vi "FTW-JSON-Core-Serialize.vi"(0 "JSON Object":i64 format="%016x", 5 "Encoding Flags":i64 format="%016x", 11 "error in":errorcluster) -> (4 "JSON Object":i64 format="%016x", 6 "JSON String (UTF-8)":string, 15 "error out":errorcluster)   [LabVIEW 2013, in "FTW-JSON.lvclass"]
uses:
  FTW-JSON.lvclass
panel:
  # "Inputs"
  # "Outputs"
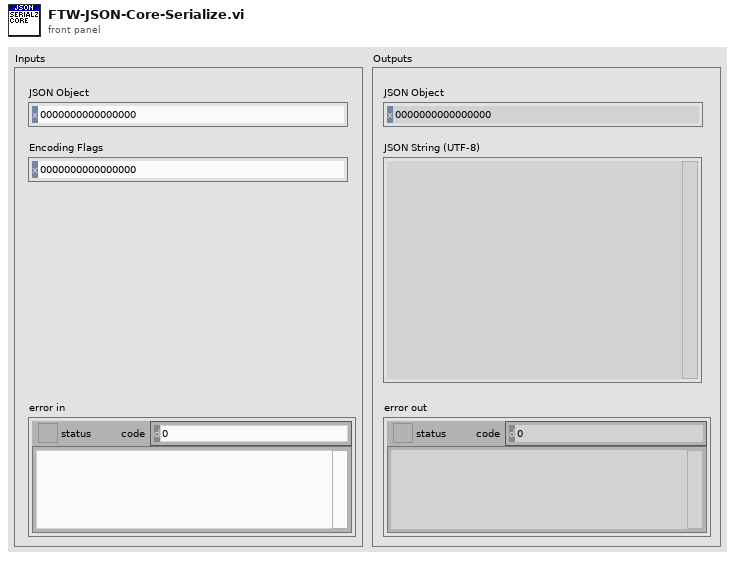
[diagram p1: front panel]
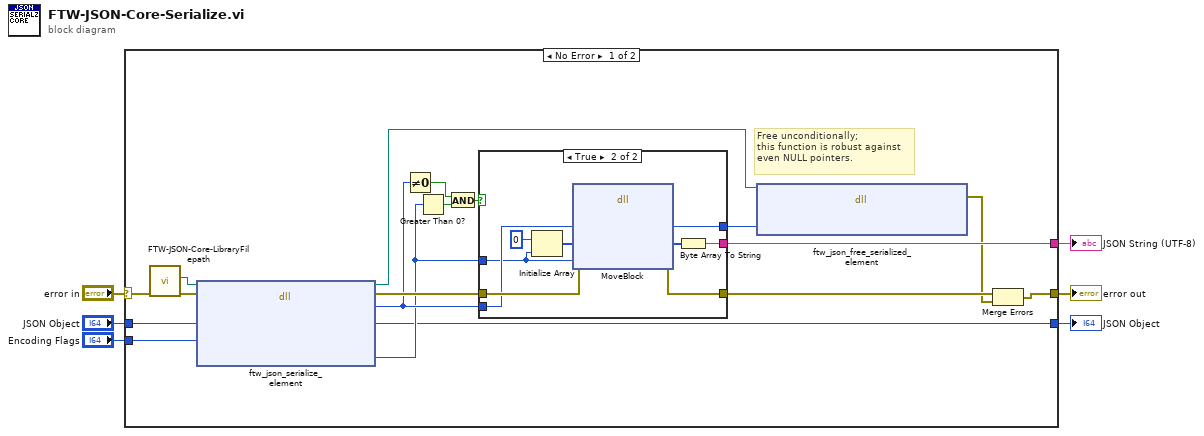
[diagram p0: block diagram]
diagram:
  n1 = case shown="No Error" "error in" {
    selector: "error in" -> [w24 w37]
    tunnel: [w23 w37] -> w6
    tunnel: [w7 w36] -> w4
    tunnel: "JSON Object" -> [w9 w36]
    tunnel: [w22 _] -> w2
    tunnel: "Encoding Flags" -> [w8 _]
    frame No Error {
      # "Free unconditionally;\nthis function is robust against\neven NULL pointers."
      n2 = call "FTW-JSON-Core-LibraryFilepath.vi"("error in"=w24) -> ("error out"=w21:errorcluster, "JSON Library Filepath"=w20:path)  [unwired: 9 in]
      n3 = dll-call lib="?" fn="ftw_json_serialize_element"(path in=w20, error in=w21, "JSON Object Pointer"=w9, "Flags"=w8) -> (path out=w10:path, error out=w19:errorcluster, "Serialized String Pointer"=w15:i64, "JSON Object Pointer"=w7:i64, "Serialized String Length"=w14:i32)  [unwired: 3 in]
      n4 = Not Equal To 0?(x=w15) -> (x != 0?=w16:bool)
      n5 = Greater Than 0?(x=w14) -> (x > 0?=w17:bool)
      n6 = And(x=w16, y=w17) -> (x .and. y?=w11:bool)
      n7 = case shown="True" w11 {
        tunnel: [_ w35] -> w22
        tunnel: w19 -> [w25 w31]
        tunnel: [w26 w30] -> w18
        tunnel: w15 -> [w26 w29]
        tunnel: w14 -> [_ w28]
        tunnel: [w25 w27] -> w13
        frame False {
        }
        frame True {
          n8 = Initialize Array(u8 0 ("element"), w28) -> (w33:u8[])
          n9 = dll-call lib="LabVIEW" fn="MoveBlock"(error in=w31, "Source Pointer"=w29, "Destination"=w33, "Length"=w28) -> (error out=w27:errorcluster, "Source Pointer"=w30:i64, "Destination"=w32:u8[])  [unwired: 4 in, 1 out]
          n10 = Byte Array To String(unsigned byte array=w32) -> (string=w35:string)
        }
      }
      n11 = dll-call lib="?" fn="ftw_json_free_serialized_element"(path in=w10, "JSON Serialized String to Free"=w18) -> (error out=w12:errorcluster)  [unwired: 4 in, 1 out]
      n12 = Merge Errors(w13, w12) -> (w23:errorcluster)
    }
    frame Error {
    }
  }
  "error out" <- w6
  "JSON Object" <- w4
  "JSON String (UTF-8)" <- w2
